vi "Node Ptr to BaseNode.vi"(8 "error in (no error)":errorcluster, 11 "nodeID in":u64) -> (0 "error out":errorcluster, 2 ".NET Refnum out":refnum<k24>, 3 "nodeID out":u64)   [LabVIEW 2019, in "TimingDRV System Explorer.lvlib"]
uses:
  TimingDRV System Explorer.lvlib
  NationalInstruments.VeriStand.SystemDefinitionAPI
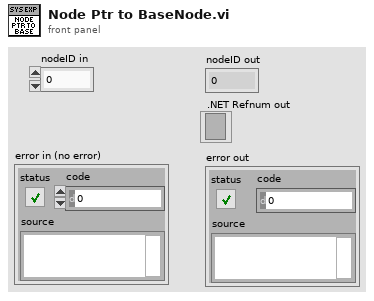
[diagram p1: front panel]
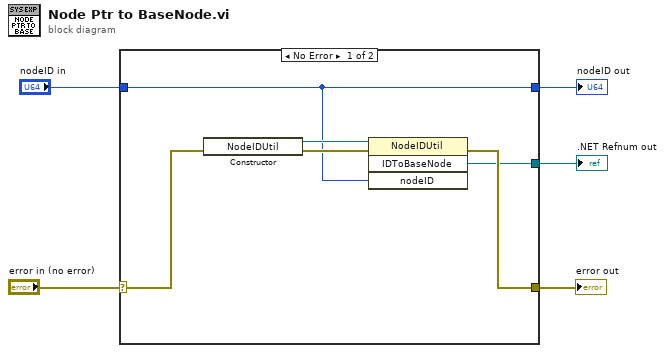
[diagram p0: block diagram]
diagram:
  n1 = case shown="No Error" "error in (no error)" {
    selector: "error in (no error)" -> [w8 w12]
    tunnel: "nodeID in" -> [w7 w13]
    tunnel: [w6 _] -> w4
    tunnel: [w10 w12] -> w3
    tunnel: [w7 w13] -> w1
    frame No Error {
      n2 = constructor class="NodeIDUtil"(error in=w8) -> (reference out=w11:refnum<k24>, error out=w9:errorcluster)  [unwired: 2 in, 1 out]
      n3 = invoke class="NodeIDUtil" method="IDToBaseNode"(reference=w11, error in=w9, "nodeID"=w7) -> (error out=w10:errorcluster, "IDToBaseNode"=w6:refnum<k24>)  [unwired: 1 in, 2 out]
    }
    frame Error {
    }
  }
  ".NET Refnum out" <- w4
  "nodeID out" <- w1
  "error out" <- w3
